vi "fix handle type.vi"(8 "error in (no error)":errorcluster, 11 "CLF Nodes":refnum<vi>[](array[refnum])) -> (0 "error out":errorcluster, 3 "Array":refnum<vi>[](array[refnum]))   [LabVIEW 2023]
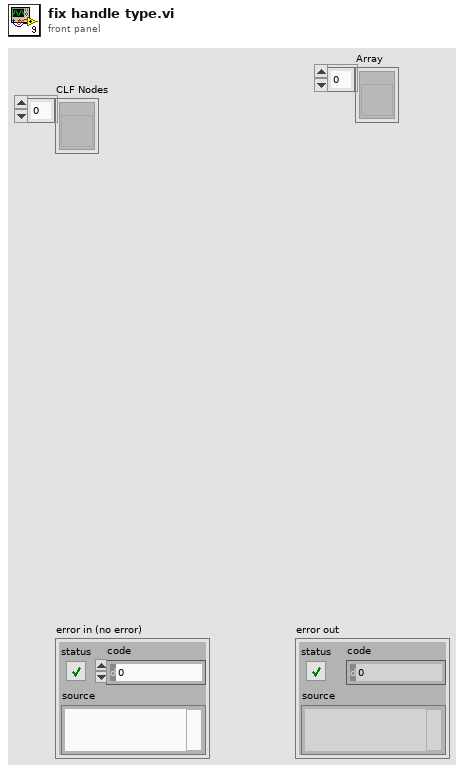
[diagram p1: front panel]
types:
  T1 = enum16{"I8", "I16", "I32", "I64", "U8", "U16", "U32", "U64", "SGL", "DBL", "PTR INT", "PTR UINT"}
  T2 = cluster{"Parameter Name":string, "Num Dimensions":i32, "Parameter Type":enum16{"Numeric", "Array", "String", "Waveform", "Digital Waveform", "Digital Table", "ActiveX", "Any", "Instance Data Pointer", "Void"}, "Numeric Type":enum16{"I8", "I16", "I32", "I64", "U8", "U16", "U32", "U64", "SGL", "DBL", "PTR INT", "PTR UINT"}, "Param Passing":enum16{"By Value", "Pointer To Value"}, "Array Passing":enum16{"Array Data Pointer", "Array Handle", "Array Handle Pointer"}, "String Passing":enum16{"C String Pointer", "Pascal String Pointer", "String Handle", "String Handle Pointer"}, "Adapt Format":enum16{"By Value", "Pointer To Value"}, "ActiveX Types":enum16{"ActiveX Variant Pointer", "IDispatch* Pointer", "IUnknown* Pointer"}, "Const (unused)":bool, "Minimum Size":string}[]
  T3 = cluster{"Parameter Name":string, "Num Dimensions":i32, "Parameter Type":enum16{"Numeric", "Array", "String", "Waveform", "Digital Waveform", "Digital Table", "ActiveX", "Any", "Instance Data Pointer", "Void"}, "Numeric Type":enum16{"I8", "I16", "I32", "I64", "U8", "U16", "U32", "U64", "SGL", "DBL", "PTR INT", "PTR UINT"}, "Param Passing":enum16{"By Value", "Pointer To Value"}, "Array Passing":enum16{"Array Data Pointer", "Array Handle", "Array Handle Pointer"}, "String Passing":enum16{"C String Pointer", "Pascal String Pointer", "String Handle", "String Handle Pointer"}, "Adapt Format":enum16{"By Value", "Pointer To Value"}, "ActiveX Types":enum16{"ActiveX Variant Pointer", "IDispatch* Pointer", "IUnknown* Pointer"}, "Const (unused)":bool, "Minimum Size":string}
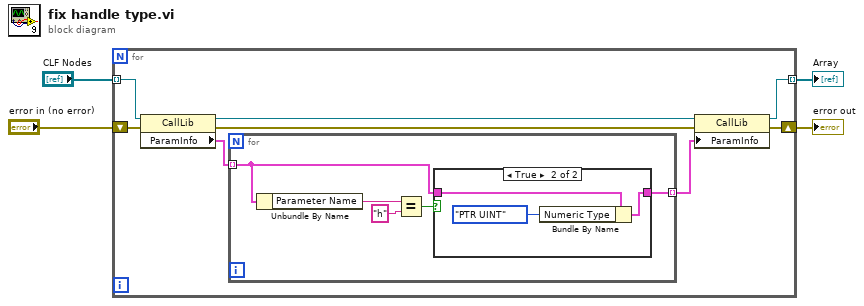
[diagram p0: block diagram]
diagram:
  n1 = for {
    shift-right: [w6] -> w4
    shift-left: "error in (no error)" -> [w11]
    tunnel: "CLF Nodes" -> [w12] mode=indexing
    tunnel: [w5] -> w1 mode=indexing
    n2 = property class="CallLib"(reference=w12, error in=w11) -> (reference out=w9:refnum<vi>, error out=w7:errorcluster, "ParamInfo"=w10:T2)
    n3 = for {
      tunnel: w10 -> [w14] mode=indexing
      tunnel: [w13] -> w8 mode=indexing
      n4 = Unbundle By Name(w14) -> ("Parameter Name"=w17:string)
      n5 = Equal?(x=w17, y="h") -> (x = y?=w15:bool)
      n6 = case shown="True" w15 {
        tunnel: w14 -> [w18 w21]
        tunnel: [w18 w19] -> w13
        frame False {
        }
        frame True {
          n7 = Bundle By Name(cluster=w21, "Numeric Type"=T1."PTR UINT") -> (w19:T3)
        }
      }
    }
    n8 = property class="CallLib"(reference=w9, error in=w7, "ParamInfo"=w8) -> (reference out=w5:refnum<vi>, error out=w6:errorcluster)
  }
  "error out" <- w4
  "Array" <- w1
